vi "coords_real_to_image_currentview.vi"(7 "Position (real coords)":cluster{"X":dbl, "Y":dbl, "Z":dbl}) -> (1 "Position (pixels, relative to the top left of the image)":cluster{dbl, dbl}, 4 "z (real coords)":dbl)   [LabVIEW 2019]
doc: "This VI converts between 'real coordinates', which are relative to the zero order spot and in metres, and pixel coordinates, relative to the top left of the current image (as produced by the VI 'anaglyph_from_scratch.vi'). There are various different views possible for the stereo system, and you can either specify manually or use the global variable (recommended) to pick the appropriate coordinate transformation(s)."
uses:
  red_tweezers_globals_INTERNAL.vi
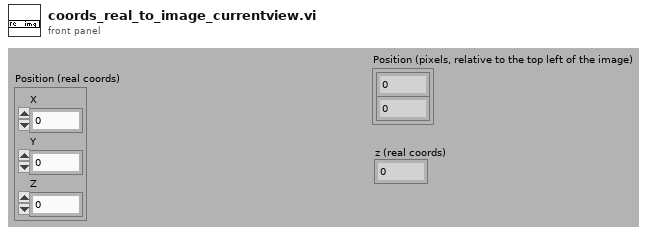
[diagram p1: front panel]
types:
  T1 = cluster{"Global ROI[0]":i32, "Global ROI[1]":i32}
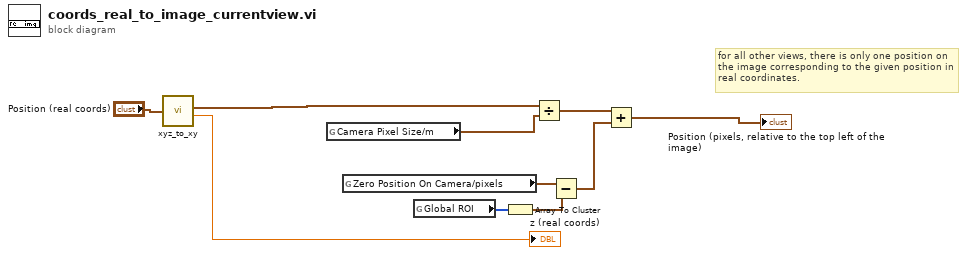
[diagram p0: block diagram]
diagram:
  # "for all other views, there is only one position on the image corresponding to the given position in real coordinates."
  n1 = call "xyz_to_xy.vi"("Position"="Position (real coords)") -> ("Position (2D)"=w5:cluster{"x":dbl, "y":dbl}, "z"=→"z (real coords)":dbl)  [unwired: 6 in]
  n2 = global read "red_tweezers_globals_INTERNAL.vi" "Camera Pixel Size/m"() -> (w9:cluster{dbl, dbl})
  n3 = global read "red_tweezers_globals_INTERNAL.vi" "Zero Position On Camera/pixels"() -> (w6:cluster{"X":dbl, "Y":dbl})
  n4 = global read "red_tweezers_globals_INTERNAL.vi" "Global ROI"() -> (w3:i32[])
  n5 = Array To Cluster(array=w3) -> (cluster=w1:T1)
  n6 = Divide(x=w5, y=w9) -> (x/y=w10:cluster{dbl, dbl})
  n7 = Subtract(x=w6, y=w1) -> (x-y=w2:cluster{dbl, dbl})
  n8 = Add(x=w10, y=w2) -> (x+y=→"Position (pixels, relative to the top left of the image)":cluster{dbl, dbl})
